vi "Build_Header_RT.vi"(9 "All_Bundled_Data_Brass":T1, 10 "ERD Number Array In":string[](array[string]), 11 "ERD Name Array In":string[](array[string])) -> (2 "ERD Name Array out 2":string[][](array[string]))   [LabVIEW 2021]
uses:
  Controls/All_Bundled_Data_RT.ctl
  Dryer Tool (Commercial 2)/JL Dryer Tool Support/type defs/Version.ctl
  Dryer Tool (Commercial 2)/JL Dryer Tool Support/type defs/ERD_Always_Show_JL.ctl
  Dryer Tool (Commercial 2)/JL Dryer Tool Support/type defs/CSV_File_String_Arrays.ctl
  Dryer Tool (Commercial 2)/JL Dryer Tool Support/type defs/Fault Table Array.ctl
  Dryer Tool (Commercial 2)/JL Dryer Tool Support/type defs/Fault_Table_Info.ctl
  Dryer Tool (Commercial 2)/JL Dryer Tool Support/type defs/BootloaderVersion.ctl
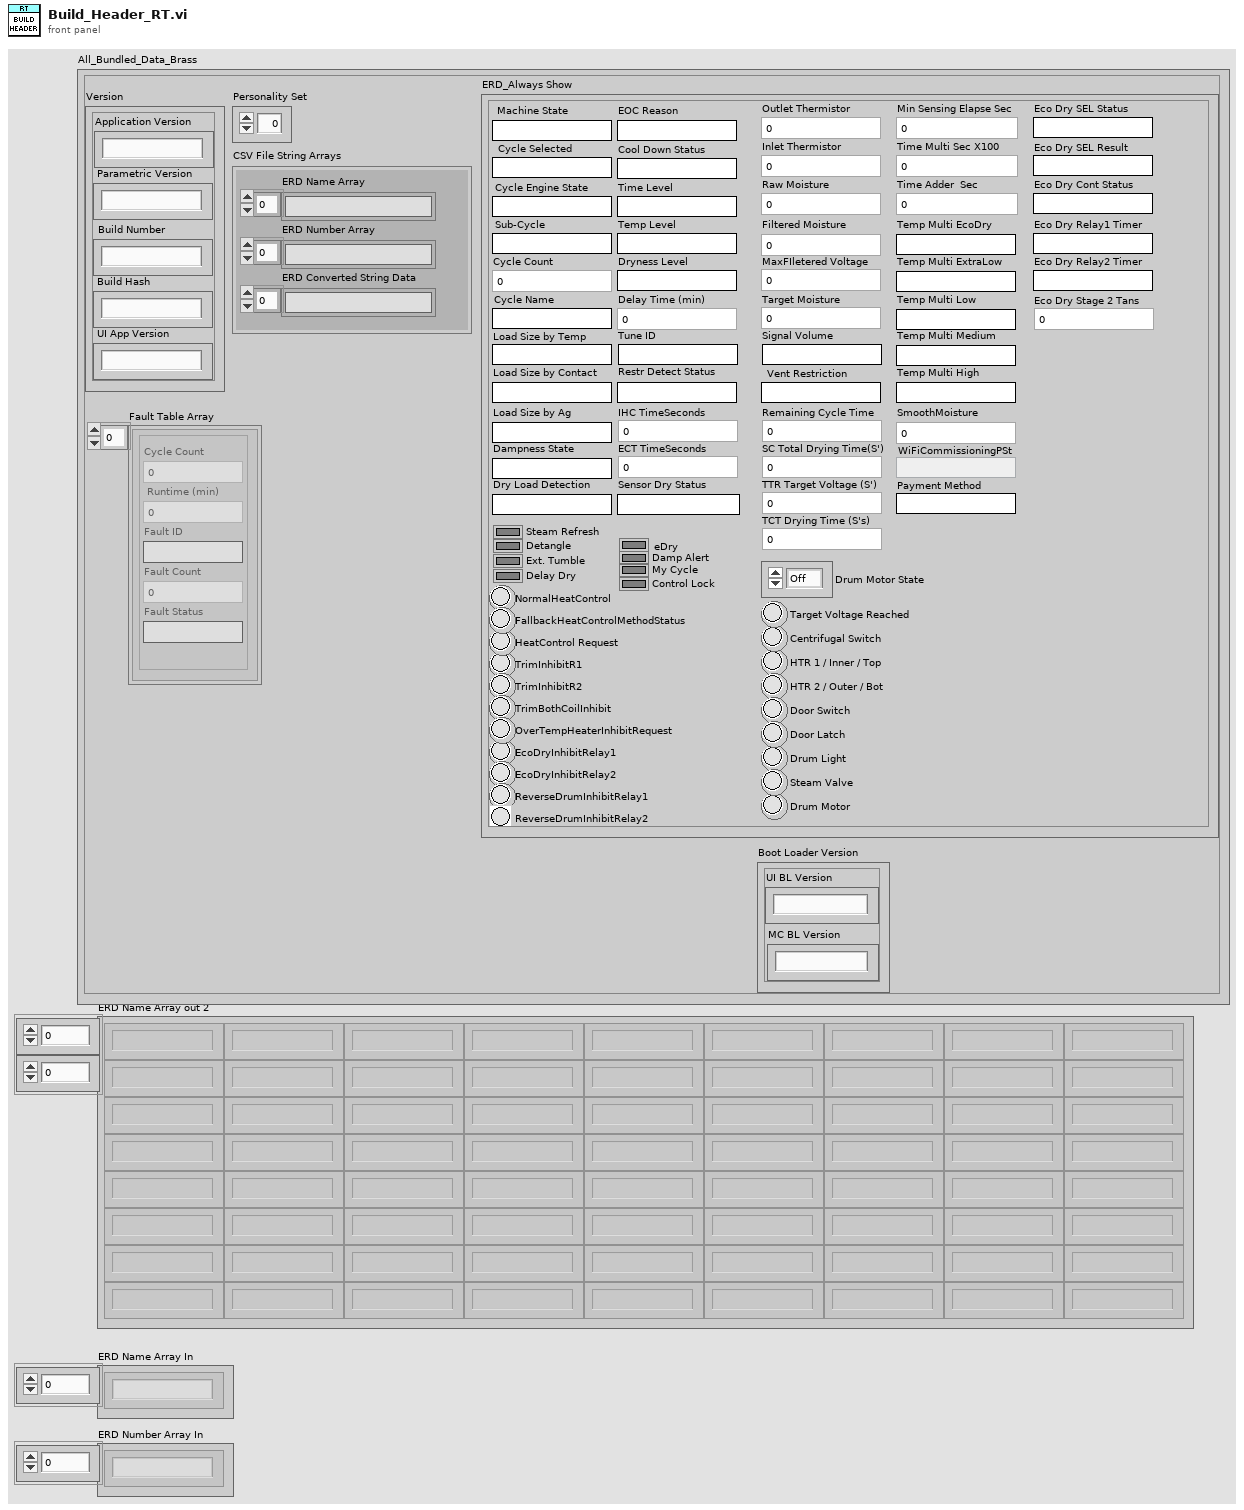
[diagram p1: front panel]
types:
  T1 = typedef "All_Bundled_Data_RT.ctl" = cluster{"Version":T2, "ERD_Always Show":T3, "Personality Set":u8, "CSV File String Arrays":T4, "Fault Table Array ":T5, "Boot Loader Version":T7}
  T2 = typedef "Version.ctl" = cluster{"Build Number":string, "Build Hash ":string, "Application Version":string, "Parametric Version":string, "UI App Version":string}
  T3 = typedef "ERD_Always_Show_JL.ctl" = cluster{"Inlet Thermistor":u16, "Machine State":string, "Filtered Moisture":u16, "Cycle Selected":string, "HTR 1 / Inner / Top":bool, "HTR 2 / Outer / Bot":bool, "Door Switch":bool, "Drum Light":bool, "Cycle Engine State":string, "Centrifugal Switch":bool, "Drum Motor":bool, "Cycle Count":u32, "Ext. Tumble":bool, "eDry":bool, "Temp Level":string, "Dryness Level":string, "Time Level":string, "Delay Time (min)":u16, "Steam Refresh":bool, "Damp Alert":bool, "Sub-Cycle":string, "Outlet Thermistor":u16, "Target Moisture":u16, "Remaining Cycle Time":u32, "Raw Moisture":u16, "Cycle Name":string, "My Cycle":bool, "Delay Dry":bool, "Detangle":bool, "Control Lock":bool, "Steam Valve":bool, "Door Latch":bool, "Signal Volume":string, "Tune ID":string, "Restr Detect Status":string, "Vent Restriction":string, "Load Size by Contact":string, "Load Size by Temp":string, "EOC Reason":string, "Sensor Dry Status":string, "Dampness State":string, "Target Voltage Reached":bool, "TrimInhibitR1":bool, "TrimInhibitR2":bool, "TrimBothCoilInhibit":bool, "NormalHeatControl":bool, "HeatControl Request":bool, "Cool Down Status":string, "EcoDryInhibitRelay1":bool, "EcoDryInhibitRelay2":bool, "ReverseDrumInhibitRelay1":bool, "ReverseDrumInhibitRelay2":bool, "OverTempHeaterInhibitRequest":bool, "FallbackHeatControlMethodStatus":bool, "IHC TimeSeconds":u32, "ECT TimeSeconds ":u32, "SC Total Drying Time(S')":u32, "TTR Target Voltage (S')":u32, "TCT Drying Time (S's)":u32, "Drum Motor State":enum16{"Off", "Cw", "Ccw", "Max"}, "Load Size by Ag":string, "MaxFIletered Voltage":u16, "Dry Load Detection":string, "Min Sensing Elapse Sec":u32, "Time Multi Sec X100":u32, "Time Adder  Sec":u32, "Temp Multi EcoDry":string, "Temp Multi ExtraLow":string, "Temp Multi Low ":string, "Temp Multi Medium":string, "Temp Multi High":string, "SmoothMoisture":u16, "Eco Dry SEL Status":string, "Eco Dry SEL Result":string, "Eco Dry Cont Status":string, "Eco Dry Relay1 Timer":string, "Eco Dry Relay2 Timer ":string, "Eco Dry Stage 2 Tans ":u32, "WiFiCommissioningPSt":string, "Payment Method":string}
  T4 = typedef "CSV_File_String_Arrays.ctl" = cluster{"ERD Number Array":string[], "ERD Name Array":string[], "ERD Converted String Data":string[]}
  T5 = typedef "Fault Table Array.ctl" = T6[]
  T6 = typedef "Fault_Table_Info.ctl" = cluster{"Cycle Count":u32, " Runtime (min) ":u32, "Fault Status":string, "Fault ID":string, "Fault Count":u16}
  T7 = typedef "BootloaderVersion.ctl" = cluster{"UI BL Version":string, "MC BL Version":string}
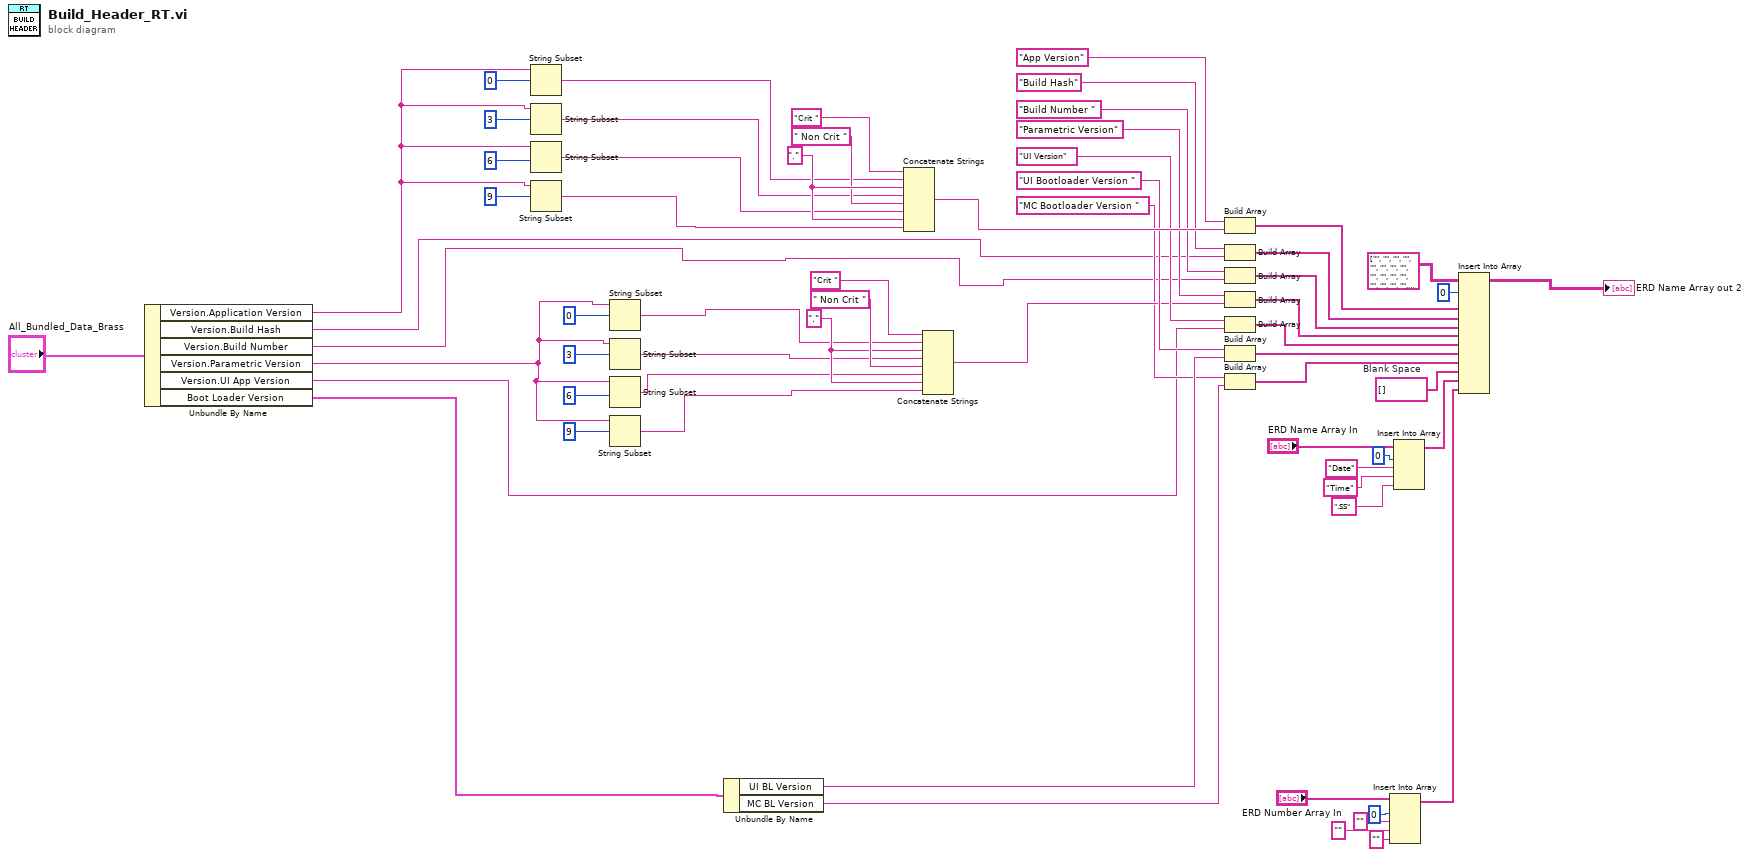
[diagram p0: block diagram]
diagram:
  w27 = string[] []  # Blank Space
  w58 = "." ("element")
  w63 = "." ("element")
  n1 = Unbundle By Name("All_Bundled_Data_Brass") -> ("Version.Application Version"=w19:string, "Version.Build Hash"=w10:string, "Version.Build Number"=w9:string, "Version.Parametric Version"=w8:string, "Version.UI App Version"=w3:string, "Boot Loader Version"=w2:T7)
  n2 = String Subset(string=w19, offset (0)=0 ("length (rest)")) -> (substring=w18:string)  [unwired: 1 in]
  n3 = String Subset(string=w19, offset (0)=3 ("length (rest)")) -> (substring=w17:string)  [unwired: 1 in]
  n4 = String Subset(string=w19, offset (0)=6) -> (substring=w16:string)  [unwired: 1 in]
  n5 = String Subset(string=w19, offset (0)=9) -> (substring=w15:string)  [unwired: 1 in]
  n6 = String Subset(string=w8, offset (0)=0 ("length (rest)")) -> (substring=w7:string)  [unwired: 1 in]
  n7 = String Subset(string=w8, offset (0)=3 ("length (rest)")) -> (substring=w6:string)  [unwired: 1 in]
  n8 = String Subset(string=w8, offset (0)=6) -> (substring=w5:string)  [unwired: 1 in]
  n9 = String Subset(string=w8, offset (0)=9) -> (substring=w4:string)  [unwired: 1 in]
  n10 = Unbundle By Name(w2) -> ("UI BL Version"=w38:string, "MC BL Version"=w28:string)
  n11 = Concatenate Strings("Crit " ("element"), w18, w63, w17, " Non Crit " ("element"), w16, w63, w15) -> (w54:string)
  n12 = Concatenate Strings("Crit " ("element"), w7, w58, w6, " Non Crit " ("element"), w5, w58, w4) -> (w37:string)
  n13 = Build Array("App Version" ("new element/subarray"), w54) -> (w56:string[])
  n14 = Build Array("Build Hash" ("new element/subarray"), w10) -> (w52:string[])
  n15 = Build Array("Build Number " ("new element/subarray"), w9) -> (w50:string[])
  n16 = Build Array("Parametric Version" ("new element/subarray"), w37) -> (w49:string[])
  n17 = Build Array("UI Version" ("new element/subarray"), w3) -> (w48:string[])
  n18 = Build Array("UI Bootloader Version " ("new element/subarray"), w38) -> (w36:string[])
  n19 = Build Array("MC Bootloader Version " ("new element/subarray"), w28) -> (w24:string[])
  n20 = Insert Into Array(array="ERD Number Array In", index=0, new element #1="" ("new element/subarray"), new element #2="" ("new element/subarray"), new element #3="" ("new element/subarray")) -> (w25:string[])
  n21 = Insert Into Array(array="ERD Name Array In", index=0, new element #1="Date", new element #2="Time", new element #3=".SS" ("new element/subarray")) -> (w26:string[])
  n22 = Insert Into Array(array=string[][] [["", "", "", "", "", "", "", "", "", "", "", "", "", "", "", "", "", "", "", "", "", "", "", "", "", "", "", "", "", "", "", "", "", "", "", "", "", "", "", "", "0"]] ("Array Ini"), index (row)=0, new element #1=w56, new element #2=w52, new element #3=w50, new element #4=w49, new element #5=w48, new element #6=w36, new element #7=w24, new element #8=w27, new element #9=w26, new element #10=w25) -> (→"ERD Name Array out 2":string[][])  [unwired: 1 in]
